vi "maxigauge_get_p.vi"(5 "maxi_delay 3":u32=500, 6 "err_in":errorcluster, 7 "maxi_delay":u32=500, 8 "maxi_delay 2":u32=500, 9 "?":i32, 10 "maxi_visa":refnum<visa-resource-name>) -> (0 "err_out":errorcluster, 3 "Pressure (Torr)":string)   [LabVIEW 2019]
panel:
  out "Overall Status":bool
  out "Acknowledgement Status":bool
  out "maxi_visa 2":refnum<visa-resource-name>
  in  "maxi_b2r 2":u32
  in  "maxi_b2r":u32
  # "Sensor Number"
  # "VISA"
  # "DELAY"
  # "BYTE AT PORT"
  # "STATUS"
  # "ERROR"
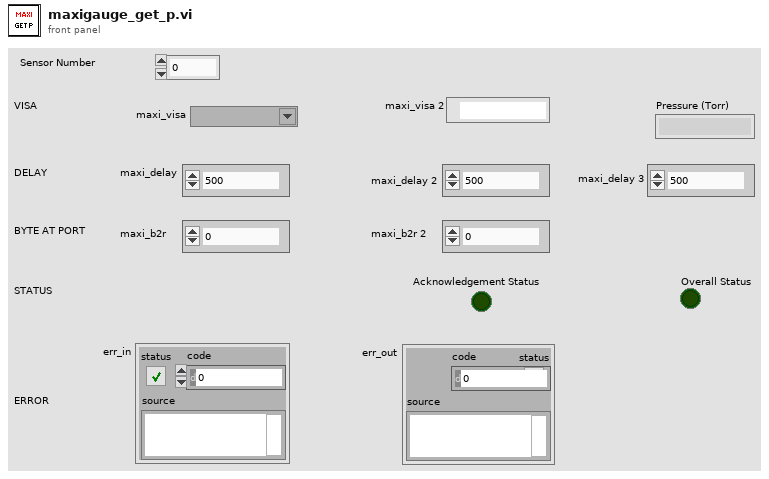
[diagram p1: front panel]
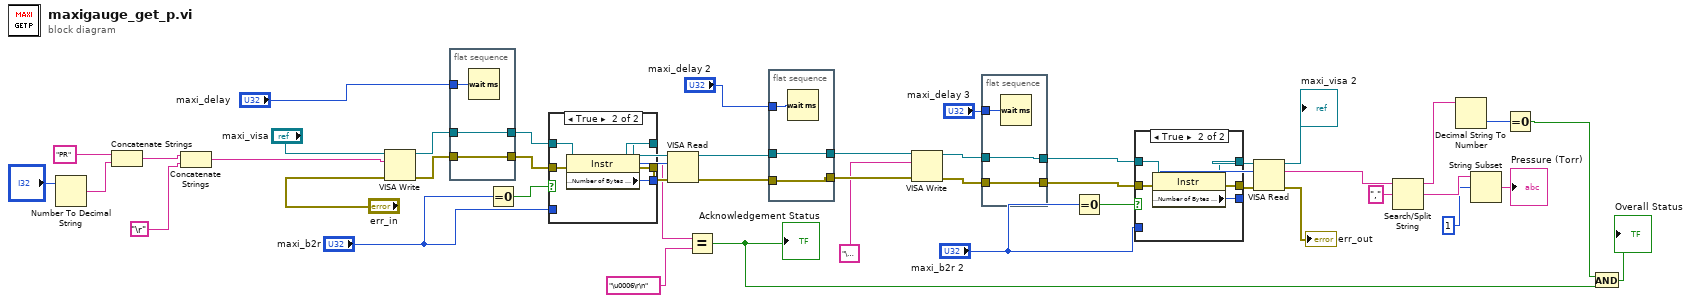
[diagram p0: block diagram]
diagram:
  n1 = Number To Decimal String(number="?") -> (decimal integer string=w2:string)  [unwired: 1 in]
  n2 = Concatenate Strings("PR" ("string"), w2) -> (w3:string)
  n3 = Concatenate Strings(w3, "\r") -> (w20:string)
  n4 = VISA Write(VISA resource name="maxi_visa", write buffer=w20, error in (no error)="err_in") -> (VISA resource name out=w46:refnum<visa-resource-name>, error out=w48:errorcluster)  [unwired: 1 out]
  n5 = flat-sequence {
    tunnel: w48 -> [w50]
    tunnel: [w50] -> w47
    tunnel: w46 -> [w49]
    tunnel: [w49] -> w45
    tunnel: "maxi_delay" -> [w51]
    frame #0 {
      n6 = Wait (ms)(milliseconds to wait=w51) -> ()  [unwired: 1 out]
    }
  }
  n7 = Equal To 0?(x="maxi_b2r") -> (x = 0?=w41:bool)
  n8 = case shown="True" w41 {
    tunnel: w47 -> [w53 w59]
    tunnel: w45 -> [w54 w58]
    tunnel: [w54 w57] -> w39
    tunnel: [w53 w56] -> w38
    tunnel: [w52 w55] -> w37
    tunnel: "maxi_b2r" -> [w52 _]
    frame False {
    }
    frame True {
      n9 = property class="Instr"(reference=w58, error in=w59) -> (reference out=w57:refnum<visa-resource-name>, error out=w56:errorcluster, "Serial Settings:Number of Bytes at Serial Port"=w55:u32)
    }
  }
  n10 = VISA Read(VISA resource name=w39, byte count=w37, error in (no error)=w38) -> (VISA resource name out=w36:refnum<visa-resource-name>, read buffer=w10:string, error out=w35:errorcluster)  [unwired: 1 out]
  n11 = Equal?(x=w10, y="\u0006\r\n") -> (x = y?=w6:bool)
  "Acknowledgement Status" <- w6
  n12 = flat-sequence {
    tunnel: [w60] -> w33
    tunnel: w36 -> [w62]
    tunnel: [w62] -> w34
    tunnel: "maxi_delay 2" -> [w61]
    tunnel: w35 -> [w60]
    frame #0 {
      n13 = Wait (ms)(milliseconds to wait=w61) -> ()  [unwired: 1 out]
    }
  }
  n14 = VISA Write(VISA resource name=w34, write buffer="\u0005", error in (no error)=w33) -> (VISA resource name out=w26:refnum<visa-resource-name>, error out=w25:errorcluster)  [unwired: 1 out]
  n15 = flat-sequence {
    tunnel: [w64] -> w32
    tunnel: [w65] -> w31
    tunnel: w26 -> [w65]
    tunnel: w25 -> [w64]
    tunnel: "maxi_delay 3" -> [w63]
    frame #0 {
      n16 = Wait (ms)(milliseconds to wait=w63) -> ()  [unwired: 1 out]
    }
  }
  n17 = Equal To 0?(x="maxi_b2r 2") -> (x = 0?=w30:bool)
  n18 = case shown="True" w30 {
    tunnel: w32 -> [w67 w73]
    tunnel: w31 -> [w68 w72]
    tunnel: [w68 w71] -> w29
    tunnel: [w67 w70] -> w28
    tunnel: [w66 w69] -> w27
    tunnel: "maxi_b2r 2" -> [w66 _]
    frame False {
    }
    frame True {
      n19 = property class="Instr"(reference=w72, error in=w73) -> (reference out=w71:refnum<visa-resource-name>, error out=w70:errorcluster, "Serial Settings:Number of Bytes at Serial Port"=w69:u32)
    }
  }
  n20 = VISA Read(VISA resource name=w29, byte count=w27, error in (no error)=w28) -> (VISA resource name out=→"maxi_visa 2":refnum<visa-resource-name>, read buffer=w18:string, error out=→"err_out":errorcluster)  [unwired: 1 out]
  n21 = Search/Split String(string=w18, search string/char (-)=",") -> (substring before match=w13:string, match + rest of string=w16:string)  [unwired: 1 in, 1 out]
  n22 = Decimal String To Number(string=w13) -> (number=w12:i32)  [unwired: 2 in, 1 out]
  n23 = String Subset(string=w16, offset (0)=1) -> (substring=→"Pressure (Torr)":string)  [unwired: 1 in]
  n24 = Equal To 0?(x=w12) -> (x = 0?=w7:bool)
  n25 = And(x=w7, y=w6) -> (x .and. y?=→"Overall Status":bool)
